vi "Query Multi Eval Meas List Segment Transform Precoding.vi"(6 "Segment (1)":T1=1, 7 "Bandwidth Part (BWP0)":i32(ring) items=["BWP0"], 8 "error in (no error)":errorcluster, 9 "Carrier Component (1)":T2=1, 10 "Instance (1)":T3=1, 11 "VISA resource name":refnum<visa-resource-name>) -> (0 "error out":errorcluster, 2 "Enabled":bool=TRUE, 3 "VISA resource name out":refnum<visa-resource-name>)   [LabVIEW 2015, in "Rohde&Schwarz CMXP NR FR2 Measurement.lvlib"]
doc: "Queries whether the <BWP> on carrier <cc> in segment <no> uses a transform precoding function.\n\nAttribute:\n-\n\nRemote-control command:\nCONFigure:NRMMw:MEAS<i>:LIST:SEGMent<no>[:CC<cc>]:BWPart:PUSCh:DFTPrecoding?"
uses:
  <instrlib>/Rohde&Schwarz CMXP NR FR2 Measurement/Rohde&Schwarz CMXP NR FR2 Measurement.lvlib
  <instrlib>/Rohde&Schwarz CMXP NR FR2 Measurement/Private/_Instance.ctl
  <instrlib>/Rohde&Schwarz CMXP NR FR2 Measurement/Private/_Carrier Component.ctl
  <instrlib>/Rohde&Schwarz CMXP NR FR2 Measurement/Private/_Segment.ctl
  <instrlib>/Rohde&Schwarz CMXP NR FR2 Measurement/Private/rsidr_core.llb/rsidr_core.lvlib
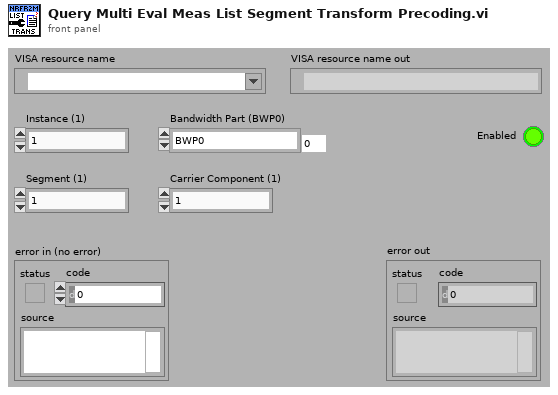
[diagram p1: front panel]
types:
  T1 = typedef "Rohde&Schwarz CMXP NR FR2 Measurement.lvlib/_Segment.ctl" = i32
  T2 = typedef "Rohde&Schwarz CMXP NR FR2 Measurement.lvlib/_Carrier Component.ctl" = i32
  T3 = typedef "Rohde&Schwarz CMXP NR FR2 Measurement.lvlib/_Instance.ctl" = i32
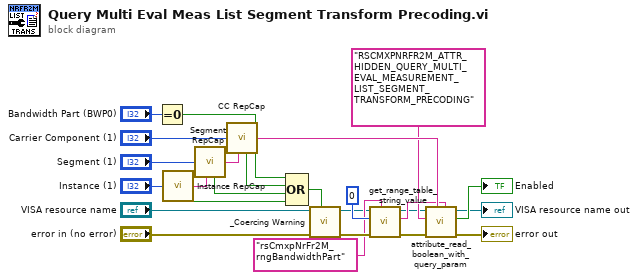
[diagram p0: block diagram]
diagram:
  n1 = Equal To 0?(x="Bandwidth Part (BWP0)") -> (x = 0?=w3:bool)
  n2 = call <instrlib>:"Instance RepCap.vi"("Instance In"="Instance (1)") -> ("In Range?"=w21:bool, "RepCap Identifier Out"=w1:string)  [unwired: 1 in]
  n3 = call <instrlib>:"Segment RepCap.vi"("Segment In"="Segment (1)", "RepCap String In (\"\")"=w1) -> ("In Range?"=w6:bool, "RepCap Identifier Out"=w4:string)
  n4 = call <instrlib>:"CC RepCap.vi"("CC In"="Carrier Component (1)", "RepCap String In (\"\")"=w4) -> ("In Range?"=w5:bool, "RepCap Identifier Out"=w16:string)
  n5 = Compound Arithmetic op=OR(w3, w5, w6, w21) -> (w22:bool)
  n6 = call <instrlib>:"_Coercing Warning.vi"("In Range?"=w22, "error in (no error)"="error in (no error)", "VISA resource name"="VISA resource name") -> ("error out"=w19:errorcluster, "VISA resource name out"=w9:refnum<visa-resource-name>)  [unwired: 7 in]
  n7 = call <instrlib>:"get_range_table_string_value.vi"("Range Table ID in"="rsCmxpNrFr2M_rngBandwidthPart", "error in"=w19, "I32 input"=0, "VISA resource name"=w9) -> ("error out"=w17:errorcluster, "String Value out"=w15:string, "VISA resource name out"=w8:refnum<visa-resource-name>)  [unwired: 5 in]
  n8 = call <instrlib>:"attribute_read_boolean_with_query_param.vi"("Query Parameter (None)"=w15, "Repeated Capability"=w16, "error in"=w17, "Attribute ID"="RSCMXPNRFR2M_ATTR_HIDDEN_QUERY_MULTI_EVAL_MEASUREMENT_LIST_SEGMENT_TRANSFORM_PRECODING", "VISA resource name"=w8) -> ("error out"=→"error out":errorcluster, "Boolean out"=→"Enabled":bool, "VISA resource name out"=→"VISA resource name out":refnum<visa-resource-name>)  [unwired: 4 in]
